vi "Set Cell .NET.vi"(10 "Cell .NET":refnum<k24>, 11 "Cell in":refnum<class "Cell.lvclass">) -> (3 "Cell out":refnum<class "Cell.lvclass">)   [LabVIEW 2024, in "SourceGrid.lvlib" / "Cell.lvclass"]
uses:
  Cell.lvclass
  D:/git/Sourcegrid-LabVIEW/dll/SourceGrid.dll
  dll/SourceGrid.dll
  Cell.lvclass/Cell.ctl
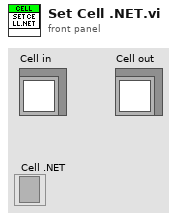
[diagram p1: front panel]
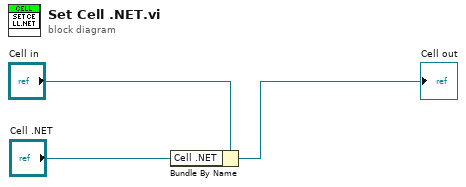
[diagram p0: block diagram]
diagram:
  n1 = Bundle By Name(cluster="Cell in", "Cell .NET"="Cell .NET") -> (→"Cell out":refnum<class "Cell.lvclass">)
